vi "Arduino Slave Addressing.vi"() -> ()   [LabVIEW 2018]
uses:
  Underlying VI's/I2C Master VI/Arduino_Interfacing.ctl
  Underlying VI's/I2C Master VI/I2C_MASTER_WRITE_NEW Type Def.ctl
panel:
  out "error out":errorcluster
  out "Arduino Data":T1
  in  "Radio Buttons":T2(radio)
  in  "stop":bool
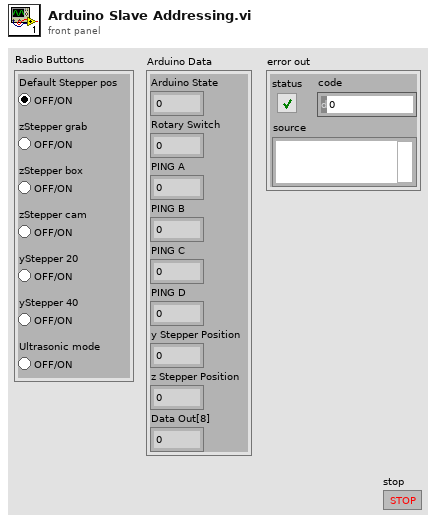
[diagram p1: front panel]
types:
  T1 = cluster{"Arduino State":u8, "Rotary Switch":u8, "PING A":u8, "PING B":u8, "PING C":u8, "PING D":u8, "y Stepper Position":u8, "z Stepper Position":u8, "Data Out[8]":u8}
  T2 = enum32{"Default Stepper pos", "zStepper grab", "zStepper box", "zStepper cam", "yStepper 20", "yStepper 40", "Ultrasonic mode"}
  T3 = typedef "Arduino_Interfacing.ctl" = enum16{"Initialize", "Write to Arduino", "Read From Arduino"}
  T4 = typedef "I2C_MASTER_WRITE_NEW Type Def.ctl" = enum16{"Ultrasonic sensors", "Stepper origin", "zStepper 13.3k", "zStepper 13k", "zStepper 12k", "zStepper 11k", "zStepper 10k", "zStepper 9k", "zStepper 8k", "zStepper 7k", "zStepper 6k", "zStepper 5k", "zStepper 4k", "zStepper 3k", "zStepper 2k", "zStepper 1k", "zStepper 900", "zStepper 800", "zStepper 700", "zStepper 600", "zStepper 500", "zStepper 400", "zStepper 300", "zStepper 200", "zStepper 100", "zStepper 0", "yStepper control", "Open Claw", "Close Claw", "Soft Reset"}
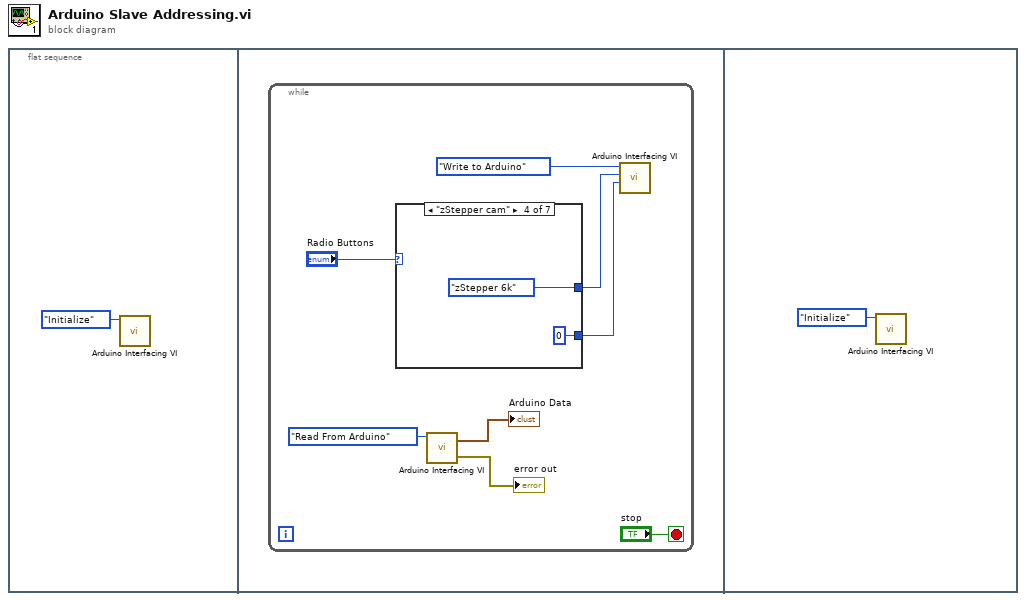
[diagram p0: block diagram]
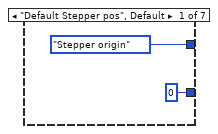
[diagram p2: hidden frame]
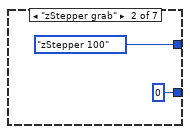
[diagram p3: hidden frame]
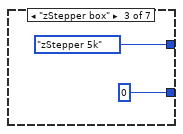
[diagram p4: hidden frame]
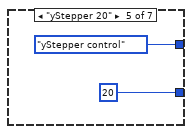
[diagram p5: hidden frame]
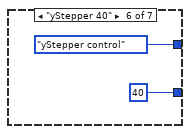
[diagram p6: hidden frame]
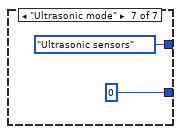
[diagram p7: hidden frame]
diagram:
  n1 = flat-sequence {
    frame #0 {
      n2 = call "Arduino Interfacing VI.vi"("AE Mode"=Arduino_Interfacing."Initialize") -> ()  [unwired: 3 in, 2 out]
    }
    frame #1 {
      n3 = while {
        stop <- "stop" stop-if-true
        n4 = case shown="\"zStepper cam\"" "Radio Buttons" {
          tunnel: [I2C_MASTER_WRITE_NEW_Type_Def."Stepper origin" ("Data to Write") I2C_MASTER_WRITE_NEW_Type_Def."zStepper 100" ("Data to Write") I2C_MASTER_WRITE_NEW_Type_Def."zStepper 5k" ("Data to Write") I2C_MASTER_WRITE_NEW_Type_Def."zStepper 6k" ("Data to Write") I2C_MASTER_WRITE_NEW_Type_Def."yStepper control" ("Data to Write") I2C_MASTER_WRITE_NEW_Type_Def."yStepper control" ("Data to Write") I2C_MASTER_WRITE_NEW_Type_Def."Ultrasonic sensors" ("Data to Write")] -> w3
          tunnel: [u8 0 ("y Stepper value") u8 0 ("y Stepper value") u8 0 ("y Stepper value") u8 0 ("y Stepper value") u8 20 ("y Stepper value") u8 40 ("y Stepper value") u8 0 ("y Stepper value")] -> w2
          frame "Default Stepper pos", Default {
          }
          frame "zStepper grab" {
          }
          frame "zStepper box" {
          }
          frame "zStepper cam" {
          }
          frame "yStepper 20" {
          }
          frame "yStepper 40" {
          }
          frame "Ultrasonic mode" {
          }
        }
        n5 = call "Arduino Interfacing VI.vi"("AE Mode"=Arduino_Interfacing."Read From Arduino") -> ("error out"=→"error out":errorcluster, "Arduino Data"=→"Arduino Data":T1)  [unwired: 3 in]
        n6 = call "Arduino Interfacing VI.vi"("y Stepper value"=w2, "Data to Write"=w3, "AE Mode"=Arduino_Interfacing."Write to Arduino") -> ()  [unwired: 1 in, 2 out]
      }
    }
    frame #2 {
      n7 = call "Arduino Interfacing VI.vi"("AE Mode"=Arduino_Interfacing."Initialize") -> ()  [unwired: 3 in, 2 out]
    }
  }
